vi "array_diff.vi"(1 "Normalized Template":dbl[](array[numeric]), 2 "In":dbl[](array[numeric])) -> (0 "Out":dbl format="%.2f")   [LabVIEW 2018]
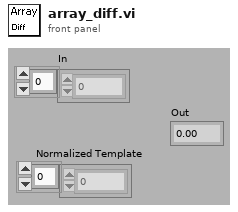
[diagram p1: front panel]
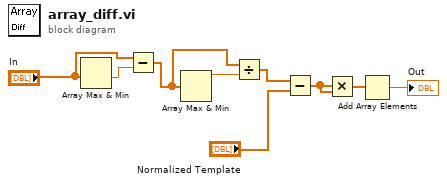
[diagram p0: block diagram]
diagram:
  n1 = Array Max & Min(array="In") -> (min value=w9:dbl)  [unwired: 3 out]
  n2 = Subtract(x="In", y=w9) -> (x-y=w8:dbl[])
  n3 = Array Max & Min(array=w8) -> (max value=w7:dbl)  [unwired: 3 out]
  n4 = Divide(x=w8, y=w7) -> (x/y=w6:dbl[])
  n5 = Subtract(x=w6, y="Normalized Template") -> (x-y=w4:dbl[])
  n6 = Multiply(x=w4, y=w4) -> (x*y=w3:dbl[])
  n7 = Add Array Elements(numeric array=w3) -> (sum=→"Out":dbl)
